vi "VI Server_M_ClmnListBox_ItemNames_SET.vi"(6 "Item Names":string[][](array[string]), 7 "Label":string, 8 "error in":errorcluster, 10 "SingleInstance":bool=TRUE, 11 "VI Server.RefsCluster":T1) -> (0 "error out":errorcluster, 1 "Multicolumn Listbox.Ref":refnum<vi>, 3 "VI Server.RefsCluster.DUP":T1)   [LabVIEW 2020]
uses:
  VI Server_TypeDefs/VI Server_RefsCluster.ctl
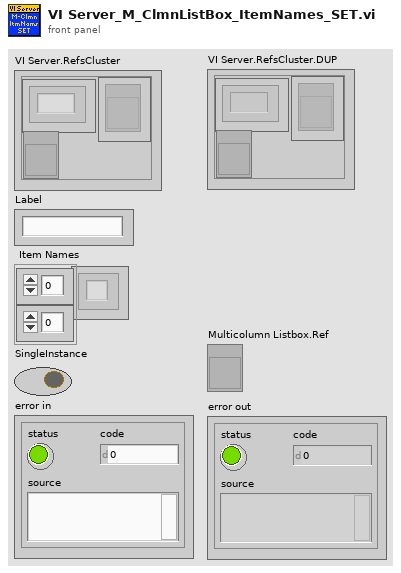
[diagram p1: front panel]
types:
  T1 = typedef "VI Server_RefsCluster.ctl" = cluster{"Labels":string[], "Refs":refnum<vi>[], "VI Ref":refnum<vi>}
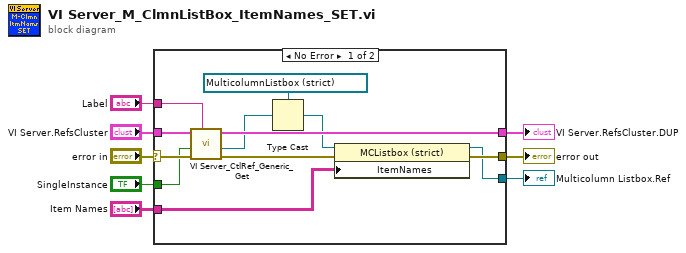
[diagram p0: block diagram]
diagram:
  n1 = case shown="No Error" "error in" {
    selector: "error in" -> [w20 w22]
    tunnel: [w11 w22] -> w7
    tunnel: "VI Server.RefsCluster" -> [w19 w21]
    tunnel: [w18 w21] -> w5
    tunnel: "Label" -> [w17 _]
    tunnel: "SingleInstance" -> [w13 _]
    tunnel: [w10 _] -> w2
    tunnel: "Item Names" -> [w9 _]
    frame No Error {
      n2 = call "VI Server_CtlRef_Generic_Get.vi"("Control.Label"=w17, "error in"=w20, "SingleInstance"=w13, "VI Server.RefsCluster"=w19) -> ("error out"=w15:errorcluster, "Control.Ref.Generic"=w16:refnum<vi>, "VI Server.RefsCluster.DUP"=w18:T1)  [unwired: 5 in]
      n3 = Type Cast(type=refnum<vi> refnum ("Multicolumn Listbox"), x=w16) -> (*(type *) &x=w14:refnum<vi>)
      n4 = property class="MCListbox (strict)"(reference=w14, error in=w15, "ItemNames"=w9) -> (reference out=w10:refnum<vi>, error out=w11:errorcluster)
    }
    frame Error {
    }
  }
  "VI Server.RefsCluster.DUP" <- w5
  "error out" <- w7
  "Multicolumn Listbox.Ref" <- w2
